vi "Get Stack ID - Answer.vi"(7 "Data":string, 8 "error in (no error)":errorcluster, 9 "Function ID":u8, 10 "Stack ID":u8, 11 "IP Connection in":refnum<class "IP Connection.lvclass">) -> (0 "error out":errorcluster, 2 "Get Stack ID Response":T1, 3 "IP Connection out":refnum<class "IP Connection.lvclass">)   [LabVIEW 2011, in "Tinkerforge.lvlib" / "IP Connection.lvclass"]
doc: "This VI interprets the <B>Get Stack ID</B> answer transfered from Brickd and sends the answer event to the requester."
uses:
  IP Connection.lvclass
  Type Definitions/Get Stack ID Response.ctl
  Device/Type Definitions/Firmware Version.ctl
  Device/Device.lvclass
  Tinkerforge.lvlib
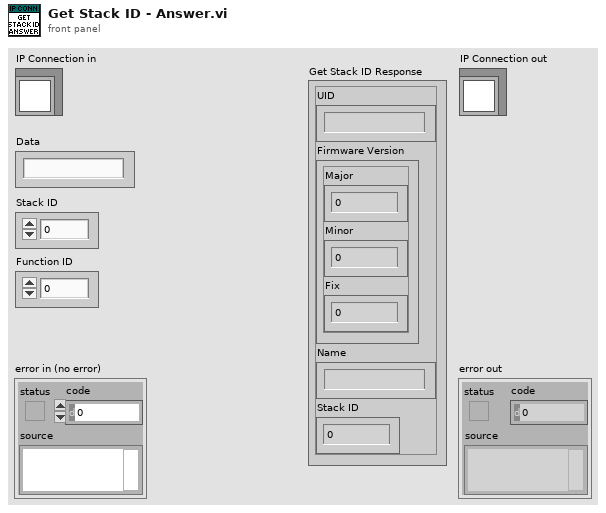
[diagram p1: front panel]
types:
  T1 = typedef "Tinkerforge.lvlib/IP Connection.lvclass/Get Stack ID Response.ctl" = cluster{"UID":string, "Firmware Version":T2, "Name":string, "Stack ID":u8}
  T2 = typedef "Tinkerforge.lvlib/Device.lvclass/Firmware Version.ctl" = cluster{"Major":u8, "Minor":u8, "Fix":u8}
  T3 = enum16{"big-endian, network order", "native, host order", "little-endian"}
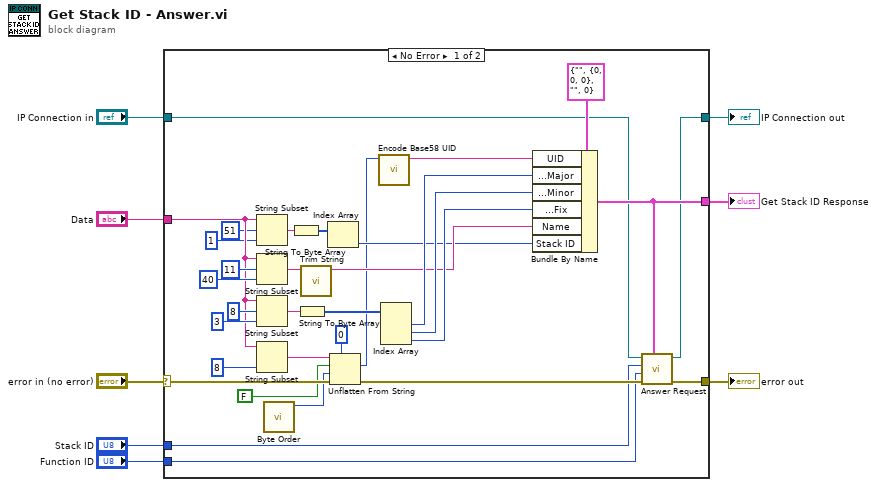
[diagram p0: block diagram]
diagram:
  n1 = case shown="No Error" "error in (no error)" {
    selector: "error in (no error)" -> [w40 w43]
    tunnel: [w16 w43] -> w7
    tunnel: [w11 w42] -> w5
    tunnel: "IP Connection in" -> [w12 w42]
    tunnel: "Data" -> [w23 _]
    tunnel: "Stack ID" -> [w14 _]
    tunnel: [w13 _] -> w2
    tunnel: "Function ID" -> [w15 _]
    frame No Error {
      n2 = String Subset(string=w23, offset (0)=51, length (rest)=1 ("length (rest)")) -> (substring=w20:string)
      n3 = String Subset(string=w23, offset (0)=11, length (rest)=40 ("length (rest)")) -> (substring=w25:string)
      n4 = String Subset(string=w23, offset (0)=8, length (rest)=3 ("length (rest)")) -> (substring=w32:string)
      n5 = String Subset(string=w23, length (rest)=8 ("length (rest)")) -> (substring=w37:string)  [unwired: 1 in]
      n6 = call "Byte Order.vi"() -> ("byte order (2:little-endian)"=w39:T3)  [unwired: 11 in]
      n7 = String To Byte Array(string=w20) -> (unsigned byte array=w19:u8[])
      n8 = String To Byte Array(string=w32) -> (unsigned byte array=w31:u8[])
      n9 = call "Trim String.vi"("String"=w25) -> ("trimmed string"=w24:string)  [unwired: 10 in]
      n10 = Index Array(array=w19) -> (element=w18:u8)  [unwired: 1 in]
      n11 = Unflatten From String(type=u64 0, binary string=w37, data includes array or string size? (T)=FALSE, byte order (0:big-endian, network order)=w39, error in (no error)=w40) -> (value=w10:u64, error out=w17:errorcluster)  [unwired: 1 out]
      n12 = call "Encode Base58 UID.vi"("UID"=w10) -> ("Base58 UID"=w9:string)  [unwired: 9 in, 1 out]
      n13 = Index Array(array=w31) -> (element #1=w30:u8, element #2=w29:u8, element #3=w28:u8)  [unwired: 3 in]
      n14 = Bundle By Name(cluster=T1 {"UID"="", "Firmware Version"={"Major"=0, "Minor"=0, "Fix"=0}, "Name"="", "Stack ID"=0} ("Get Stack ID Response"), "UID"=w9, "Firmware Version.Major"=w30, "Firmware Version.Minor"=w29, "Firmware Version.Fix"=w28, "Name"=w24, "Stack ID"=w18) -> (w13:T1)
      n15 = call "Answer Request.vi"("Data"=w13, "error in (no error)"=w17, "Function ID"=w15, "Stack ID"=w14, "IP Connection in"=w12) -> ("error out"=w16:errorcluster, "IP Connection out"=w11:refnum<class "IP Connection.lvclass">)  [unwired: 5 in]
    }
    frame Error {
    }
  }
  "error out" <- w7
  "IP Connection out" <- w5
  "Get Stack ID Response" <- w2
